vi "Test.vi"() -> ()   [LabVIEW 2018, in "ScopePlugins.lvlib" / "NIScope.lvclass"]
uses:
  NIScope.lvclass
  Shared/TypeDefs/Channel.ctl
  Shared/TypeDefs/Acquisition.ctl
  <instrlib>/niScope/Controls/niScope trigger slope.ctl
  <instrlib>/niScope/Controls/niScope acquisition type.ctl
  <instrlib>/niScope/Configure/Trigger/niScope Configure Trigger Digital.vi
  <instrlib>/niScope/Acquire/Fetch/niScope Multi Fetch Cluster.vi
  <instrlib>/niScope/Acquire/niScope Multi Read Cluster.vi
  ScopePlugins.lvlib
panel:
  out "wfm info":T1(array[cluster]) {"reserved2" format="%.2f"; "reserved1" format="%.2f"; "offset" format="%^.3e"; "gain" format="%^.3e"; "xIncrement" format="%^.3e"; "relativeInitialX" format="%^.3e"; "absoluteInitialX" format="%^.3e"}
  in  "number of records":i32=1
  out "x != 0?":bool
  out "time":dbl
  out "Sessions":refnum<k20>[](array[refnum])
  out "Fetch:Records Done":i32
  out "transposed array":dbl[][](array[numeric])
  out "wfm":dbl[][](array[numeric])
  out "Waveform Chart 2":dbl[][](graph)
  in  "Stop Button":bool
  out "Waveform Chart":waveform(dbl)[](graph)
  in  "Trigger":T2={"Coupling"=enum."DC", "Holdoff"=0.0, "Level"=0.2, "Slope"=enum."Positive", "Source"="PXI_Trig0", "Type"=enum."Edge"}
  in  "Acquisition":T3={"StartTime"=0.0, "Type"=enum."Normal", "NumPointsMin"=50000, "RecordLength"=50000, "SampleRate"=50000.0, "TimePerRecord"=0.001, "SamplingMode "=enum."Real Time", "Interpolation"=enum."No Interpolation", "NumAverages"=8, "Resolution"=enum."Auto", "EnableAveraging"=FALSE, "Continuous"=TRUE}
  out "error out":errorcluster
  in  "Channels":T4[](array[typedef])=[{"Enabled"=TRUE, "Name"="0", "InputImpedance"=1000000.0, "InputFreqMax"=0.0, "ProbeAttn"=1.0, "Coupling"=enum."DC", "Offset"=0.0, "Range"=10.0, "Handle"="PXI1Slot8", "Connected"=FALSE, "Options String "=""}, {"Enabled"=TRUE, "Name"="0", "InputImpedance"=1000000.0, "InputFreqMax"=0.0, "ProbeAttn"=1.0, "Coupling"=enum."DC", "Offset"=0.0, "Range"=10.0, "Handle"="PXI1Slot7", "Connected"=FALSE, "Options String "=""}, {"Enabled"=TRUE, "Name"="0", "InputImpedance"=1000000.0, "InputFreqMax"=0.0, "ProbeAttn"=1.0, "Coupling"=enum."DC", "Offset"=0.0, "Range"=10.0, "Handle"="PXI1Slot2", "Connected"=FALSE, "Options String "=""}]
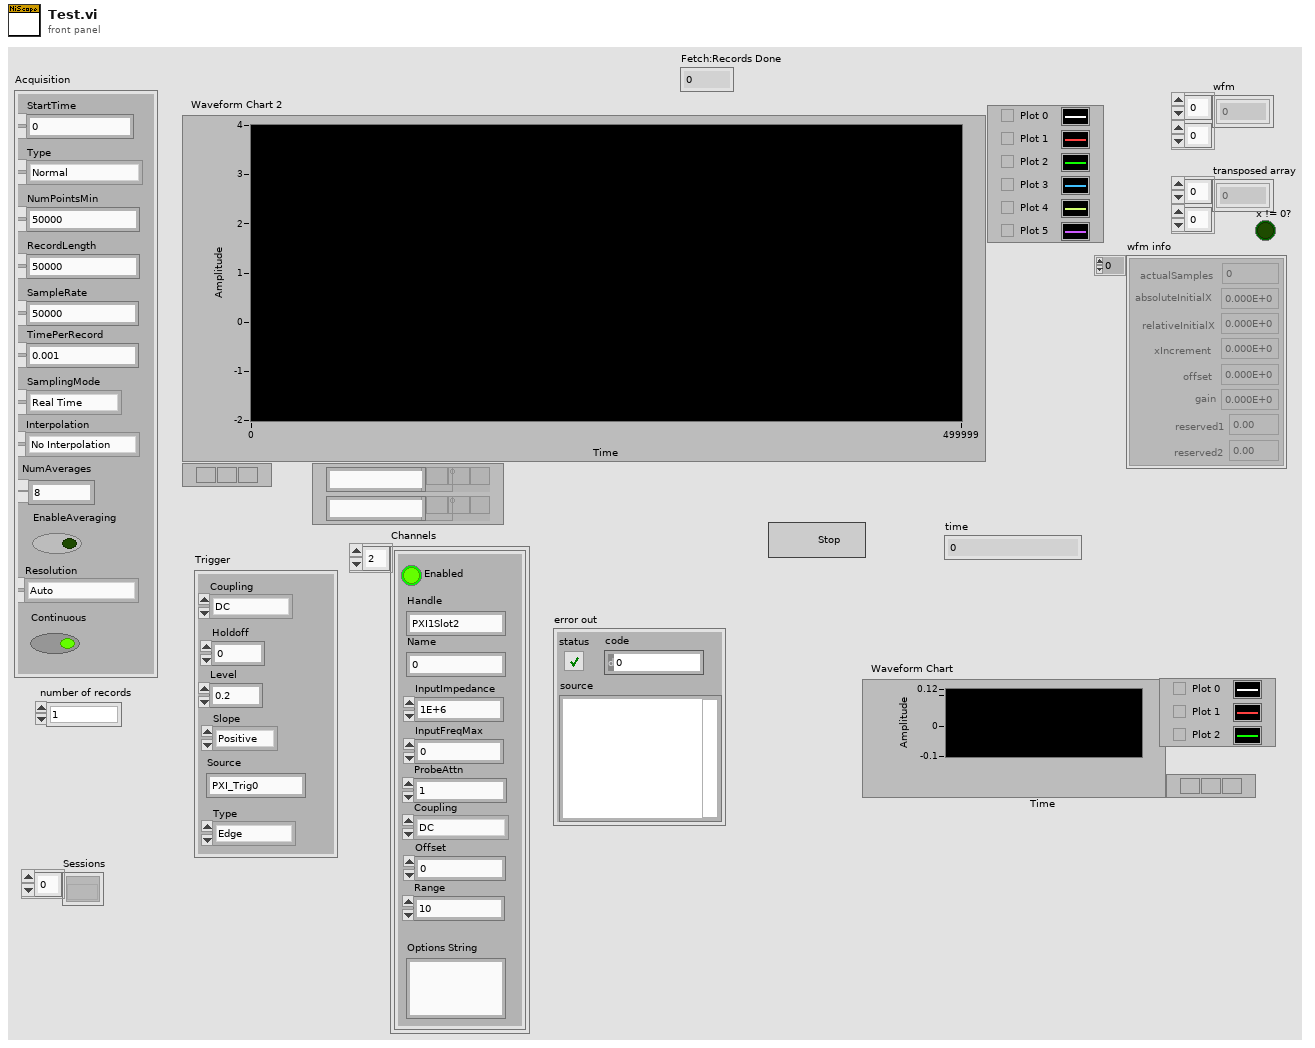
[diagram p1: front panel]
types:
  T1 = cluster{"actualSamples":i32, "absoluteInitialX":dbl, "relativeInitialX":dbl, "xIncrement":dbl, "offset":dbl, "gain":dbl, "reserved1":dbl, "reserved2":dbl}[]
  T2 = cluster{"Coupling":enum16{"AC", "DC", "LF Reject", "HF Reject", "Noise Reject"}, "Holdoff":dbl, "Level":dbl, "Slope":enum16{"Negative", "Positive"}, "Source":string, "Type":enum16{"Edge", "Width", "Runt", "Glitch", "TV", "Immediate", "AC Line"}}
  T3 = typedef "ScopePlugins.lvlib/Acquisition.ctl" = cluster{"StartTime":dbl, "Type":enum16{"Normal", "PeakDetect", "HighRes", "Envelope", "Average"}, "NumPointsMin":i32, "RecordLength":i32, "SampleRate":dbl, "TimePerRecord":dbl, "SamplingMode ":enum16{"Real Time", "Equivalent Time", "Segment", "Real Time Peak Detect", "Real Time High Resolution", "Peak Detect Segment", "High Resolution Segment"}, "Interpolation":enum16{"No Interpolation", "sin(x)/x", "linear", "1 Point sin(x)/x", "2 Point sin(x)/x", "4 Point sin(x)/x", "8 Point sin(x)/x", "16 Point sin(x)/x"}, "NumAverages":i32, "Resolution":enum16{"Auto", "Bits 9", "Bits 10", "Bits 11", "Bits 12"}, "EnableAveraging":bool, "Continuous":bool}
  T4 = typedef "ScopePlugins.lvlib/Channel.ctl" = cluster{"Enabled":bool, "Name":string, "InputImpedance":dbl, "InputFreqMax":dbl, "ProbeAttn":dbl, "Coupling":enum16{"AC", "DC", "GND"}, "Offset":dbl, "Range":dbl, "Handle":string, "Connected":bool, "Options String ":string}
  T5 = enum16{"Normal", "PeakDetect", "HighRes", "Envelope", "Average"}
  T6 = enum16{"Real Time", "Equivalent Time", "Segment", "Real Time Peak Detect", "Real Time High Resolution", "Peak Detect Segment", "High Resolution Segment"}
  T7 = typedef "niScope acquisition type.ctl" = i32
  T8 = typedef "niScope trigger slope.ctl" = i32
  T9 = cluster{"relativeInitialX":dbl, "xIncrement":dbl, "wfm":dbl[]}[]
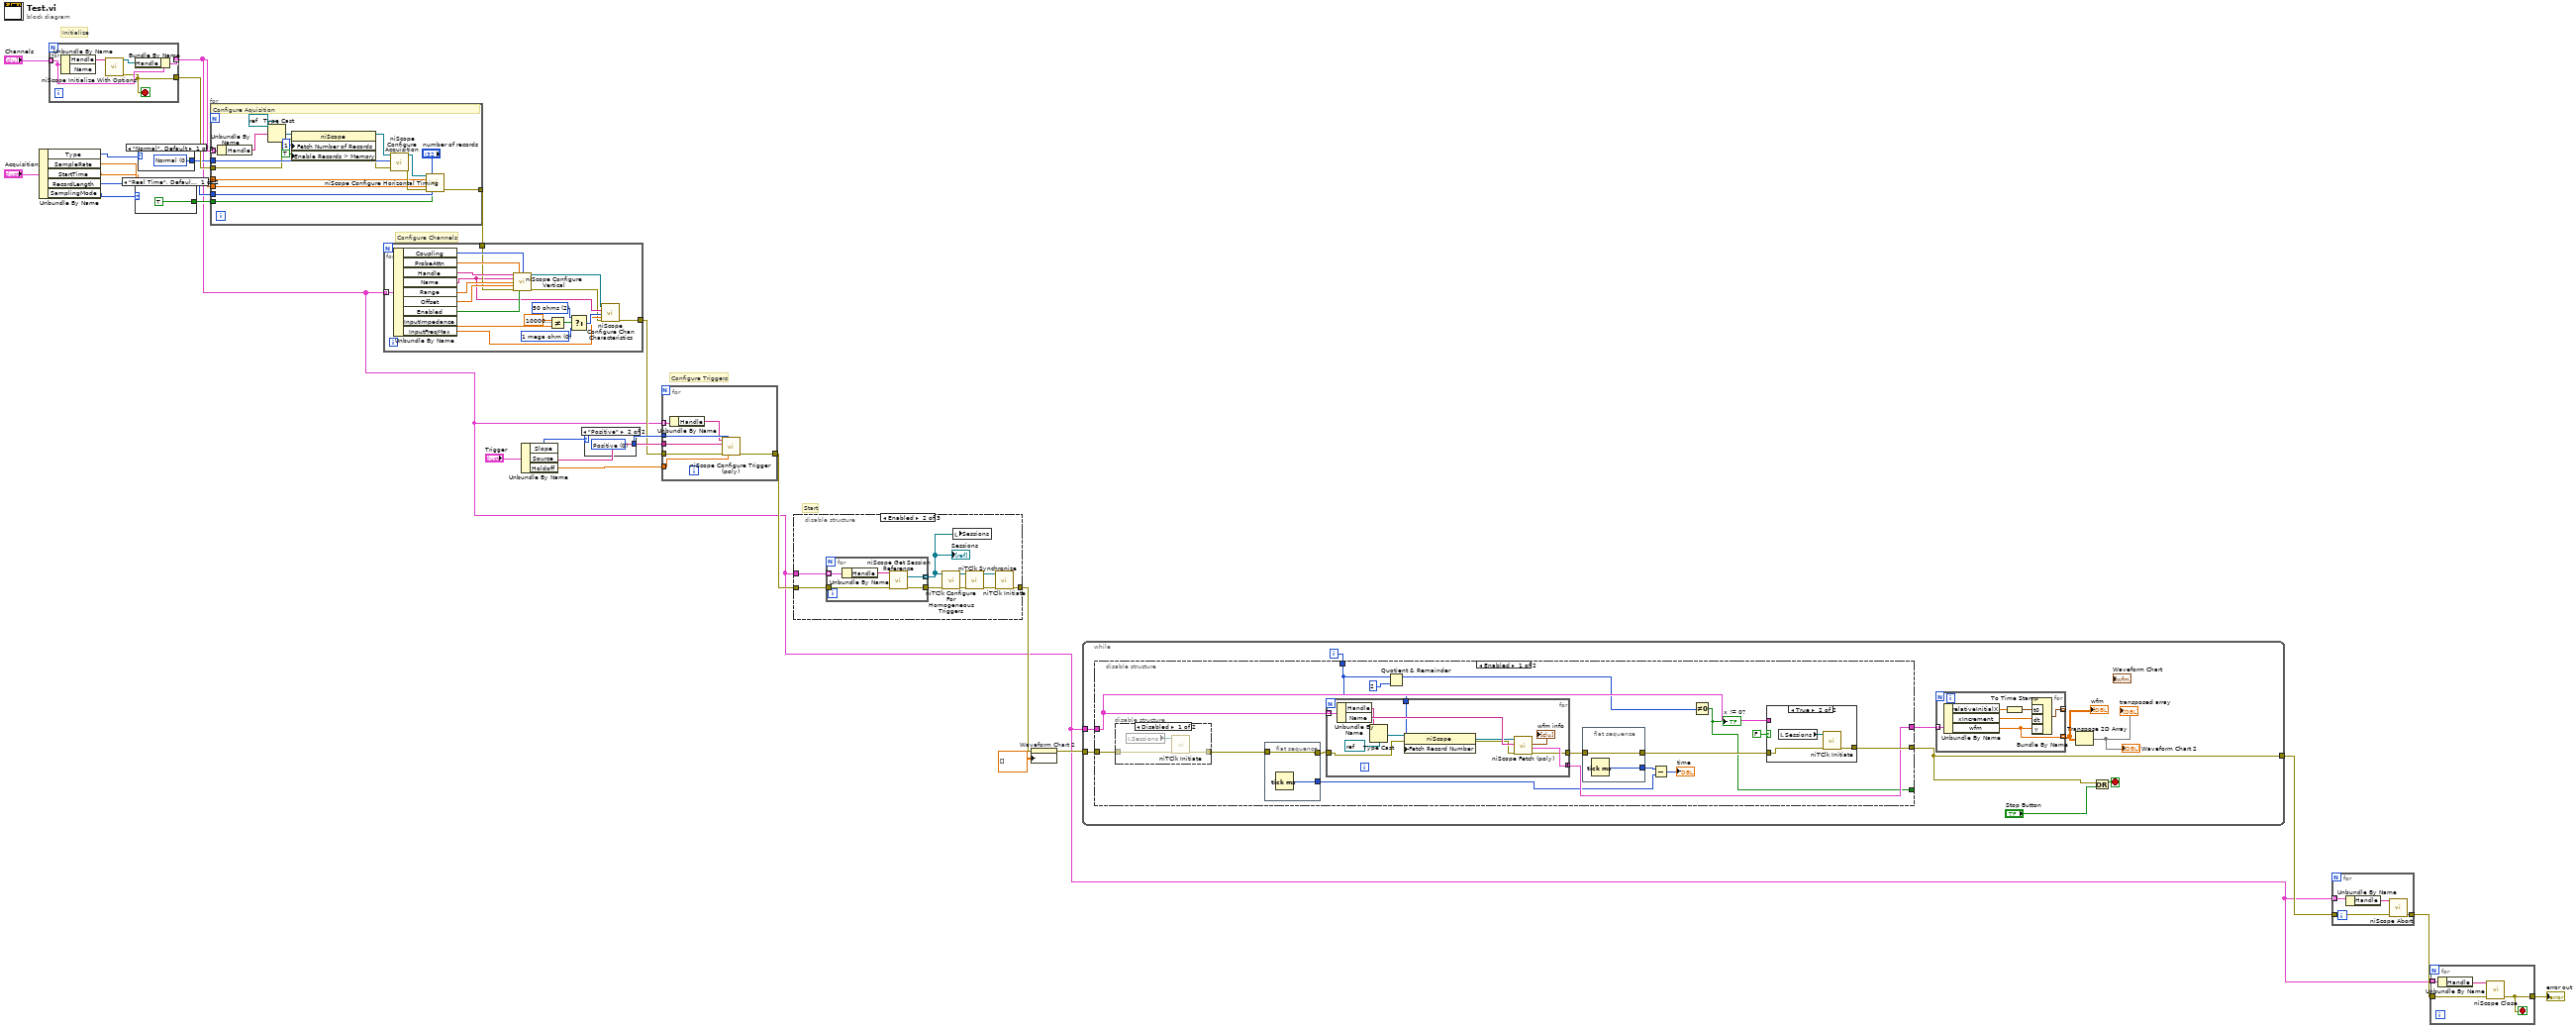
[diagram p0: block diagram]
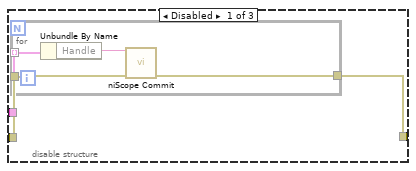
[diagram p2: hidden frame]
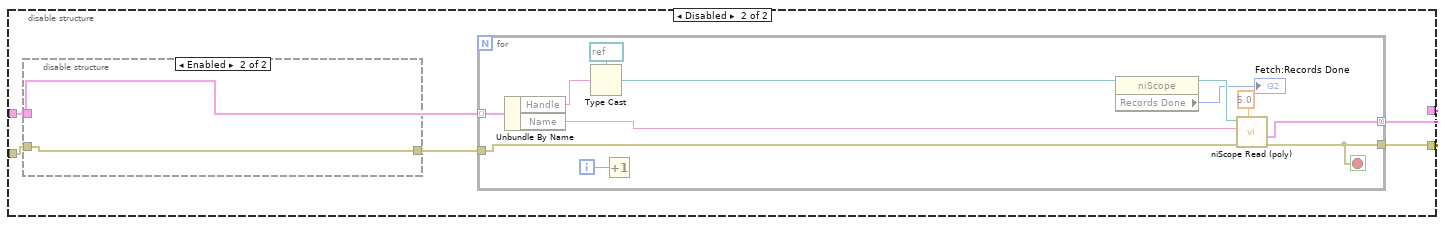
[diagram p6: hidden frame]
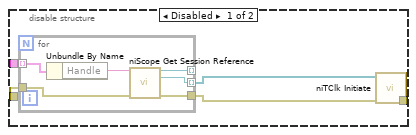
[diagram p7: hidden frame]
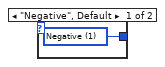
[diagram p8: hidden frame]
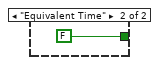
[diagram p9: hidden frame]
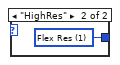
[diagram p10: hidden frame]
diagram:
  # "Start"
  # "Configure Triggers"
  # "Configure Channels"
  # "Initialize"
  n1 = Unbundle By Name("Acquisition") -> ("Type"=w22:T5, "SampleRate"=w18:dbl, "StartTime"=w17:dbl, "RecordLength"=w16:i32, "SamplingMode"=w21:T6)
  n2 = for {
    tunnel: "Channels" -> [w29] mode=indexing
    tunnel: [w26] -> w20
    tunnel: [w28] -> w1 mode=indexing
    stop <- w26 stop-if-true
    n3 = Unbundle By Name(w29) -> ("Handle"=w30:string)  [unwired: 1 out]
    n4 = call <instrlib>:"niScope Initialize With Options.vi"("resource name"=w30) -> ("instrument handle"=w27:refnum<k15>, "error out"=w26:errorcluster)  [unwired: 13 in]
    n5 = Bundle By Name(cluster=w29, "Handle"=w27) -> (w28:T4)
  }
  n6 = case shown="\"Real Time\", Default" w21 {
    tunnel: [TRUE FALSE] -> w9
    frame "Real Time", Default {
    }
    frame "Equivalent Time" {
    }
  }
  n7 = case shown="\"Normal\", Default" w22 {
    tunnel: [w33 w34] -> w19
    frame "Normal", Default {
      w33 = T7 0 items=["Normal"=0, "Flex Res"=1, "DDC"=3] ("acquisition Type")
    }
    frame "HighRes" {
      w34 = T7 1 items=["Normal"=0, "Flex Res"=1, "DDC"=3] ("acquisition Type")
    }
  }
  n8 = for {
    tunnel: w1 -> [w51] mode=indexing
    tunnel: w20 -> [w38]
    tunnel: w19 -> [w52]
    tunnel: w18 -> [w48]
    tunnel: w17 -> [w47]
    tunnel: w16 -> [w46]
    tunnel: [w35] -> w10
    tunnel: w9 -> [w45]
    # "Configure Aquisition"
    n9 = Unbundle By Name(w51) -> ("Handle"=w43:string)
    n10 = Type Cast(type=refnum<k15> refnum ("instrument handle out"), x=w43) -> (*(type *) &x=w39:refnum<k15>)
    n11 = property class="niScope"(reference=w39, error in=w38, "Fetch Number of Records"=1 ("Fetch:Fetch Number of Records"), "Enable Records > Memory"=TRUE ("Horizontal:Enable Records > Memory")) -> (reference out=w36:refnum<k15>, error out=w37:errorcluster)
    n12 = call <instrlib>:"niScope Configure Acquisition.vi"("instrument handle"=w36, "acquisition Type"=w52, "error in"=w37) -> ("instrument handle out"=w50:refnum<k15>, "error out"=w49:errorcluster)  [unwired: 11 in]
    n13 = call <instrlib>:"niScope Configure Horizontal Timing.vi"("instrument handle"=w50, "number of records"="number of records", "enforce realtime"=w45, "min sample rate"=w48, "reference position"=w47, "error in"=w49, "min record length"=w46) -> ("error out"=w35:errorcluster)  [unwired: 7 in, 1 out]
  }
  n14 = for {
    tunnel: w1 -> [w71] mode=indexing
    tunnel: w10 -> [w65]
    tunnel: [w54] -> w8
    w63 = u32 0 items=["1 mega ohm"=0, "50 ohms"=2] ("input impedance")
    w58 = u32 2 items=["1 mega ohm"=0, "50 ohms"=2] ("input impedance")
    n15 = Unbundle By Name(w71) -> ("Coupling"=w70:enum16{"AC", "DC", "GND"}, "ProbeAttn"=w69:dbl, "Handle"=w68:string, "Name"=w56:string, "Range"=w67:dbl, "Offset"=w66:dbl, "Enabled"=w64:bool, "InputImpedance"=w59:dbl, "InputFreqMax"=w57:dbl)
    n16 = call <instrlib>:"niScope Configure Vertical.vi"("instrument handle"=w68, "probe attenuation"=w69, "vertical coupling"=w70, "channels"=w56, "vertical range"=w67, "vertical offset"=w66, "error in"=w65, "channel enabled"=w64) -> ("instrument handle out"=w53:refnum<k15>, "error out"=w55:errorcluster)  [unwired: 6 in]
    n17 = Not Equal?(x=1000000.0, y=w59) -> (x != y?=w61:bool)
    n18 = Select(t=w58, s=w61, f=w63) -> (s? t:f=w60:u32)
    n19 = call <instrlib>:"niScope Configure Chan Characteristics.vi"("instrument handle"=w53, "channels"=w56, "input impedance"=w60, "maximum input frequency"=w57, "error in"=w55) -> ("error out"=w54:errorcluster)  [unwired: 9 in, 1 out]
  }
  n20 = Unbundle By Name("Trigger") -> ("Slope"=w14:enum16{"Negative", "Positive"}, "Source"=w12:string, "Holdoff"=w11:dbl)
  n21 = case shown="\"Positive\"" w14 {
    tunnel: [w72 w73] -> w13
    frame "Negative", Default {
      w72 = T8 1 items=["Positive", "Negative"] ("trigger slope")
    }
    frame "Positive" {
      w73 = T8 0 items=["Positive", "Negative"] ("trigger slope")
    }
  }
  n22 = for {
    tunnel: w13 -> [w80]
    tunnel: w12 -> [w79]
    tunnel: w11 -> [w78]
    tunnel: w8 -> [w77]
    tunnel: [w76] -> w7
    tunnel: w1 -> [w75] mode=indexing
    n23 = Unbundle By Name(w75) -> ("Handle"=w74:string)
    n24 = call-poly <instrlib>:"niScope Configure Trigger (poly).vi"("instrument handle"=w74, "trigger slope"=w80, "trigger source"=w79, "error in"=w77, "trigger holdoff"=w78) -> ("error out"=w76:errorcluster)  [unwired: 9 in, 1 out]
  }
  n25 = disable-structure shown="Enabled" {
    disable-tunnel: w7 -> [w83 w96 w102]
    disable-tunnel: [w82 w90 w102] -> w3
    disable-tunnel: w1 -> [w81 w95 _]
    frame Disabled {
      n26 = for {
        tunnel: w81 -> [w87] mode=indexing
        tunnel: w83 -> [w85]
        tunnel: [w84] -> w82
        n27 = Unbundle By Name(w87) -> ("Handle"=w86:string)
        n28 = call <instrlib>:"niScope Commit.vi"("instrument handle"=w86, "error in"=w85) -> ("error out"=w84:errorcluster)  [unwired: 12 in, 1 out]
      }
    }
    frame Enabled {
      n29 = for {
        tunnel: [w101] -> w88 mode=indexing
        tunnel: [w100] -> w94
        tunnel: w95 -> [w99] mode=indexing
        tunnel: w96 -> [w97]
        n30 = Unbundle By Name(w99) -> ("Handle"=w98:string)
        n31 = call <instrlib>:"niScope Get Session Reference.vi"("instrument handle"=w98, "error in"=w97) -> ("session reference"=w101:refnum<k20>, "error out"=w100:errorcluster)  [unwired: 11 in, 1 out]
      }
      "Sessions" <- w88
      n32 = call <instrlib>:"niTClk Configure For Homogeneous Triggers.vi"("error in (no error)"=w94, "sessions"=w88) -> ("error out"=w93:errorcluster, "sessions out"=w92:refnum<k20>[])  [unwired: 8 in]
      n33 = local write "Sessions"(w88) -> ()
      n34 = call <instrlib>:"niTClk Synchronize.vi"("error in (no error)"=w93, "sessions"=w92) -> ("error out"=w91:errorcluster, "sessions out"=w89:refnum<k20>[])  [unwired: 8 in]
      n35 = call <instrlib>:"niTClk Initiate.vi"("error in (no error)"=w91, "sessions"=w89) -> ("error out"=w90:errorcluster)  [unwired: 8 in, 1 out]
    }
    frame Disabled {
    }
  }
  n36 = property on="Waveform Chart 2" class="WFChart (strict)"(error in=w3, "History Data"=dbl[][] []) -> (error out=w4:errorcluster)  [unwired: 1 in, 1 out]
  n37 = while {
    tunnel: w1 -> [w110]
    tunnel: w4 -> [w111]
    tunnel: [w105] -> w6
    i -> [w104]
    stop <- w106 stop-if-true
    n38 = disable-structure shown="Enabled" {
      disable-tunnel: w111 -> [w127 w154]
      disable-tunnel: [w126 w155] -> w105
      disable-tunnel: w110 -> [w124 w152]
      disable-tunnel: [w125 w156] -> w109
      disable-tunnel: w104 -> [w112 _]
      disable-tunnel: [w115 _] -> _
      frame Enabled {
        n39 = disable-structure shown="Disabled" {
          disable-tunnel: w127 -> [w136 w139]
          disable-tunnel: [w138 w139] -> w122
          frame Disabled {
            n40 = local read "Sessions"() -> (w137:refnum<k20>[])
            n41 = call <instrlib>:"niTClk Initiate.vi"("error in (no error)"=w136, "sessions"=w137) -> ("error out"=w138:errorcluster)  [unwired: 8 in, 1 out]
          }
          frame Enabled {
          }
        }
        n42 = flat-sequence {
          tunnel: w122 -> [w131]
          tunnel: [w131] -> w121
          tunnel: [w130] -> w117
          frame #0 {
            n43 = Tick Count (ms)() -> (millisecond timer value=w130:u32)
          }
        }
        n44 = for {
          tunnel: w121 -> [w145]
          tunnel: [w148] -> w120
          tunnel: [w149] -> w125 mode=concatenating
          tunnel: w124 -> [w151] mode=indexing
          tunnel: w112 -> [w142]
          n45 = Unbundle By Name(w151) -> ("Handle"=w144:string, "Name"=w150:string)
          n46 = Type Cast(type=refnum<k15> refnum ("instrument handle out"), x=w144) -> (*(type *) &x=w146:refnum<k15>)
          n47 = property class="niScope"(reference=w146, error in=w145, "Fetch Record Number"=w142) -> (reference out=w143:refnum<k15>, error out=w141:errorcluster)
          n48 = call-poly <instrlib>:"niScope Fetch (poly).vi"("error in"=w141, "channels"=w150, "instrument handle"=w143) -> ("error out"=w148:errorcluster, "waveform"=w149:T9, "wfm info"=→"wfm info":T1)  [unwired: 5 in, 1 out]
        }
        n49 = Quotient & Remainder(x=w112, y=2) -> (x-y*floor(x/y)=w114:i32)  [unwired: 1 out]
        n50 = flat-sequence {
          tunnel: w120 -> [w129]
          tunnel: [w129] -> w119
          tunnel: [w128] -> w118
          frame #0 {
            n51 = Tick Count (ms)() -> (millisecond timer value=w128:u32)
          }
        }
        n52 = Subtract(x=w118, y=w117) -> (x-y=→"time":u32)
        n53 = Not Equal To 0?(x=w114) -> (x != 0?=w115:bool)
        "x != 0?" <- w115
        n54 = case shown="True" FALSE {
          tunnel: w124 -> [_ _]
          tunnel: w119 -> [w132 w133]
          tunnel: [w132 w135] -> w126
          frame False {
          }
          frame True {
            n55 = local read "Sessions"() -> (w134:refnum<k20>[])
            n56 = call <instrlib>:"niTClk Initiate.vi"("error in (no error)"=w133, "sessions"=w134) -> ("error out"=w135:errorcluster)  [unwired: 8 in, 1 out]
          }
        }
      }
      frame Disabled {
        n57 = disable-structure shown="Enabled" {
          disable-tunnel: w154 -> [w161 w168]
          disable-tunnel: w152 -> [w158 _]
          disable-tunnel: [w157 w168] -> w153
          frame Disabled {
            n58 = for {
              tunnel: [w167] -> w159 mode=indexing
              tunnel: [w166] -> _ mode=indexing
              tunnel: [w165] -> w160
              tunnel: w158 -> [w164] mode=indexing
              tunnel: w161 -> [w162]
              n59 = Unbundle By Name(w164) -> ("Handle"=w163:string)
              n60 = call <instrlib>:"niScope Get Session Reference.vi"("instrument handle"=w163, "error in"=w162) -> ("instrument handle out"=w166:refnum<k15>, "session reference"=w167:refnum<k20>, "error out"=w165:errorcluster)  [unwired: 11 in]
            }
            n61 = call <instrlib>:"niTClk Initiate.vi"("error in (no error)"=w160, "sessions"=w159) -> ("error out"=w157:errorcluster)  [unwired: 8 in, 1 out]
          }
          frame Enabled {
          }
        }
        n62 = for {
          tunnel: w152 -> [w180] mode=indexing
          tunnel: [w178] -> w155
          tunnel: [w179] -> w156 mode=concatenating
          tunnel: w153 -> [w169]
          i -> [w170]
          stop <- w178 stop-if-true
          n63 = Unbundle By Name(w180) -> ("Handle"=w174:string, "Name"=w175:string)
          n64 = Type Cast(type=refnum<k15> refnum ("instrument handle"), x=w174) -> (*(type *) &x=w173:refnum<k15>)
          n65 = Increment(x=w170) -> ()  [unwired: 1 out]
          n66 = property class="niScope"(reference=w173) -> (reference out=w172:refnum<k15>, "Records Done"=→"Fetch:Records Done":i32)  [unwired: 1 in, 1 out]
          n67 = call-poly <instrlib>:"niScope Read (poly).vi"("timeout"=5.0, "error in"=w169, "channels"=w175, "instrument handle"=w172) -> ("error out"=w178:errorcluster, "waveform"=w179:T9)  [unwired: 4 in, 2 out]
        }
      }
    }
    n68 = for {
      tunnel: w109 -> [w186] mode=indexing
      tunnel: [w182] -> _ mode=indexing
      tunnel: [w181] -> w108 mode=indexing
      n69 = Unbundle By Name(w186) -> ("relativeInitialX"=w185:dbl, "xIncrement"=w183:dbl, "wfm"=w181:dbl[])
      n70 = To Time Stamp(1:w185) -> (0:w184:timestamp)
      n71 = Bundle By Name("t0"=w184, "dt"=w183, "Y"=w181) -> (w182:waveform(dbl))  [unwired: 1 in]
    }
    "wfm" <- w108
    n72 = Transpose 2D Array(2D array=w108) -> (transposed array=→"Waveform Chart 2" →"transposed array":dbl[][])
    n73 = Or(x=w105, y="Stop Button") -> (x .or. y?=w106:bool)
  }
  n74 = for {
    tunnel: w1 -> [w190] mode=indexing
    tunnel: w6 -> [w189]
    tunnel: [w187] -> w5
    n75 = Unbundle By Name(w190) -> ("Handle"=w188:string)
    n76 = call <instrlib>:"niScope Abort.vi"("instrument handle"=w188, "error in"=w189) -> ("error out"=w187:errorcluster)  [unwired: 12 in, 1 out]
  }
  n77 = for {
    tunnel: [w194] -> w24
    tunnel: w1 -> [w192] mode=indexing
    tunnel: w5 -> [w191]
    stop <- w194 stop-if-true
    n78 = Unbundle By Name(w192) -> ("Handle"=w193:string)
    n79 = call <instrlib>:"niScope Close.vi"("instrument handle"=w193, "error in"=w191) -> ("error out"=w194:errorcluster)  [unwired: 13 in]
  }
  "error out" <- w24
